vi "sub_shutdown.vi"(7 "type":T1, 8 "error in (no error)":errorcluster, 11 "completion":bool) -> (0 "error out":errorcluster)   [LabVIEW 2019]
uses:
  shutdown-type.ctl
  _ctrl/init-r-stop.ctl
  result.ctl
  SubVIs/common/hw-control.ctl
  8fb67333-444f-4712-9ef5-9737c9c6e22f.vi
  60c8f1e5-aa91-4ba2-a334-5865b9030432.vi
  2e48ccf8-daca-4025-8b5e-31ffc1ae0acd.vi
  09bc9839-f2c0-48a8-914d-692b7bae2475.vi
  _ctrl/create-rw-close.ctl
  _ctrl/start.ctl
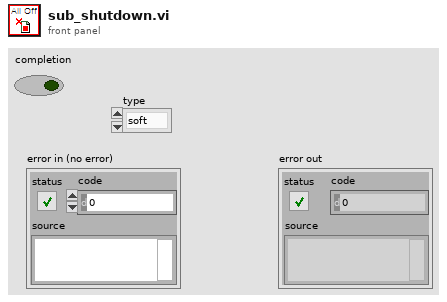
[diagram p1: front panel]
types:
  T1 = typedef "shutdown-type.ctl" = enum16{"soft", "all"}
  T2 = typedef "result.ctl" = enum16{"Init", "OK", "NG", "Shutdown", "Testing", "Completion", "Device Error", "Start", "작동", "미작동", "작동 대기", "작동 1"}
  T3 = typedef "init-r-stop.ctl" = enum16{"ini", "read", "stop"}
  T4 = typedef "hw-control.ctl" = enum16{"DL950 ready", "DL950 clear", "DL950 trigger", "DL950 read", "DL950 read seq", "DL950 Tsingle query", "AO 12v", "AO wave", "AO 0v", "relay all-off", "Discharge check", "Discharge", "Relay1", "Relay2", "Relay3", "Relay4", "Relay5", "Relay6", "BP4610 onoff", "BP4610 set", "DSP1500 set", "DSP1500 onoff"}
  T5 = typedef "start.ctl" = enum16{"init", "open", "set", "start", "stop", "read", "read_items", "query", "close", "T_single", "reset", "exit"}
  T6 = typedef "create-rw-close.ctl" = enum16{"create", "write", "read", "delete", "close"}
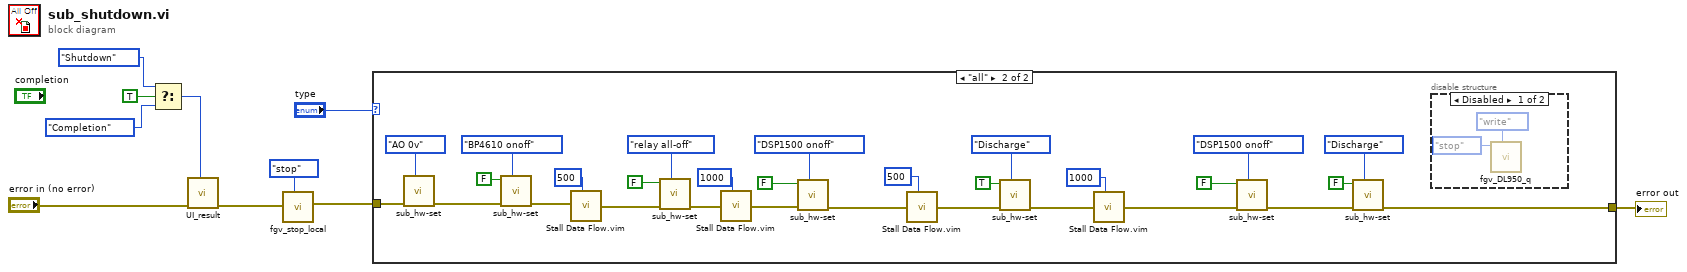
[diagram p0: block diagram]
diagram:
  n1 = Select(t=result."Shutdown", s=TRUE, f=result."Completion" ("result")) -> (s? t:f=w3:T2)
  n2 = call "UI_result.vi"("result"=w3, "error in (no error)"="error in (no error)") -> ("error out"=w5:errorcluster)  [unwired: 9 in]
  n3 = call "fgv_stop_local.vi"("cmd"=init-r-stop."stop", "error in (no error)"=w5) -> ("error out"=w9:errorcluster)  [unwired: 8 in, 1 out]
  n4 = case shown="\"all\"" "type" {
    tunnel: w9 -> [w11 w32]
    tunnel: [w11 w12] -> w7
    frame "soft", Default {
    }
    frame "all" {
      n5 = call "sub_hw-set.vi"("cmd"=hw-control."AO 0v", "error in"=w32) -> ("error out"=w33:errorcluster)  [unwired: 9 in]
      n6 = call "sub_hw-set.vi"("cmd"=hw-control."BP4610 onoff", "error in"=w33, "onoff"=FALSE) -> ("error out"=w15:errorcluster)  [unwired: 8 in]
      n7 = call "Stall Data Flow.vim"("value in"=w15, "milliseconds to wait"=u32 500 ("dt")) -> ("value out"=w14:errorcluster)  [unwired: 1 out]
      n8 = call "sub_hw-set.vi"("cmd"=hw-control."relay all-off", "error in"=w14, "onoff"=FALSE) -> ("error out"=w22:errorcluster)  [unwired: 8 in]
      n9 = call "Stall Data Flow.vim"("value in"=w22, "milliseconds to wait"=u32 1000 ("dt")) -> ("value out"=w20:errorcluster)  [unwired: 1 out]
      n10 = call "sub_hw-set.vi"("cmd"=hw-control."DSP1500 onoff", "error in"=w20, "onoff"=FALSE) -> ("error out"=w18:errorcluster)  [unwired: 8 in]
      n11 = call "Stall Data Flow.vim"("value in"=w18, "milliseconds to wait"=u32 500 ("dt")) -> ("value out"=w17:errorcluster)  [unwired: 1 out]
      n12 = call "sub_hw-set.vi"("cmd"=hw-control."Discharge", "error in"=w17, "onoff"=TRUE) -> ("error out"=w30:errorcluster)  [unwired: 8 in]
      n13 = call "Stall Data Flow.vim"("value in"=w30, "milliseconds to wait"=u32 1000 ("dt")) -> ("value out"=w27:errorcluster)  [unwired: 1 out]
      n14 = call "sub_hw-set.vi"("cmd"=hw-control."DSP1500 onoff", "error in"=w27, "onoff"=FALSE) -> ("error out"=w23:errorcluster)  [unwired: 8 in]
      n15 = call "sub_hw-set.vi"("cmd"=hw-control."Discharge", "error in"=w23, "onoff"=FALSE) -> ("error out"=w12:errorcluster)  [unwired: 8 in]
      n16 = disable-structure shown="Disabled" {
        frame Disabled {
          n17 = call "fgv_DL950_q.vi"("cmd"=create-rw-close."write", "data"=start."stop") -> ()  [unwired: 8 in, 2 out]
        }
        frame Enabled {
        }
      }
    }
  }
  "error out" <- w7
